vi "dll_newBox.vi"(8 "error in (no error)":errorcluster, 9 "height":dbl, 10 "breadth":dbl, 11 "length":dbl) -> (0 "error out":errorcluster, 3 "p_box":i32)   [LabVIEW 2020, in "box.lvlib"]
uses:
  box.lvlib
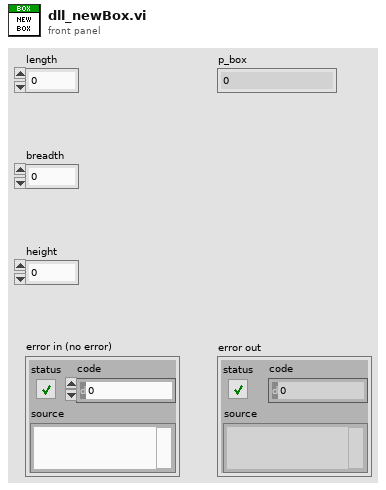
[diagram p1: front panel]
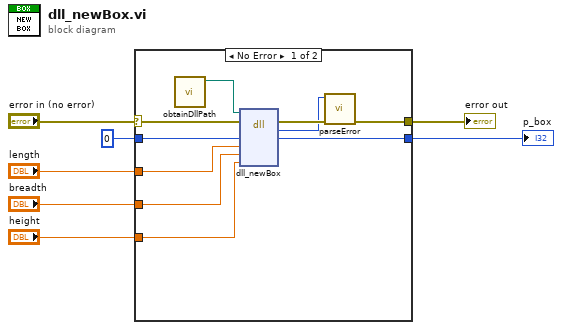
[diagram p0: block diagram]
diagram:
  n1 = case shown="No Error" "error in (no error)" {
    selector: "error in (no error)" -> [w17 w18]
    tunnel: 0 -> [w16 w19]
    tunnel: [w10 w18] -> w4
    tunnel: [w14 w19] -> w5
    tunnel: "breadth" -> [w13 _]
    tunnel: "length" -> [w12 _]
    tunnel: "height" -> [w11 _]
    frame No Error {
      n2 = call "obtainDllPath.vi"() -> ("box.dll path"=w8:path)  [unwired: 11 in]
      n3 = dll-call lib="box.dll" fn="dll_newBox"(path in=w8, error in=w17, "p_box"=w16, "length"=w12, "breadth"=w13, "height"=w11) -> (error out=w15:errorcluster, "return type"=w9:i32, "p_box"=w14:i32)  [unwired: 4 in, 1 out]
      n4 = call "parseError.vi"("error in (no error)"=w15, "status code"=w9) -> ("error out"=w10:errorcluster)  [unwired: 9 in]
    }
    frame Error {
    }
  }
  "p_box" <- w5
  "error out" <- w4
